vi "5.7.4-Forebrain_to_OCU-UDPServer.vi"() -> ()   [LabVIEW 2010]
doc: "Creates a named service and listens on the first available port. Whenever a client connects to the service, it responds with a message containing joystick data. The VI can be stopped using the STOP button."
uses:
  6-OCU Neurons/CommonIndicators.ctl
  4-High Neurons/4.4-How Sensor Typedef.ctl
  5.0-Global.vi
panel:
  out "5.7.2 Main Indicators":T1
  out "data out":string
  out "error out":errorcluster
  in  "error in":errorcluster
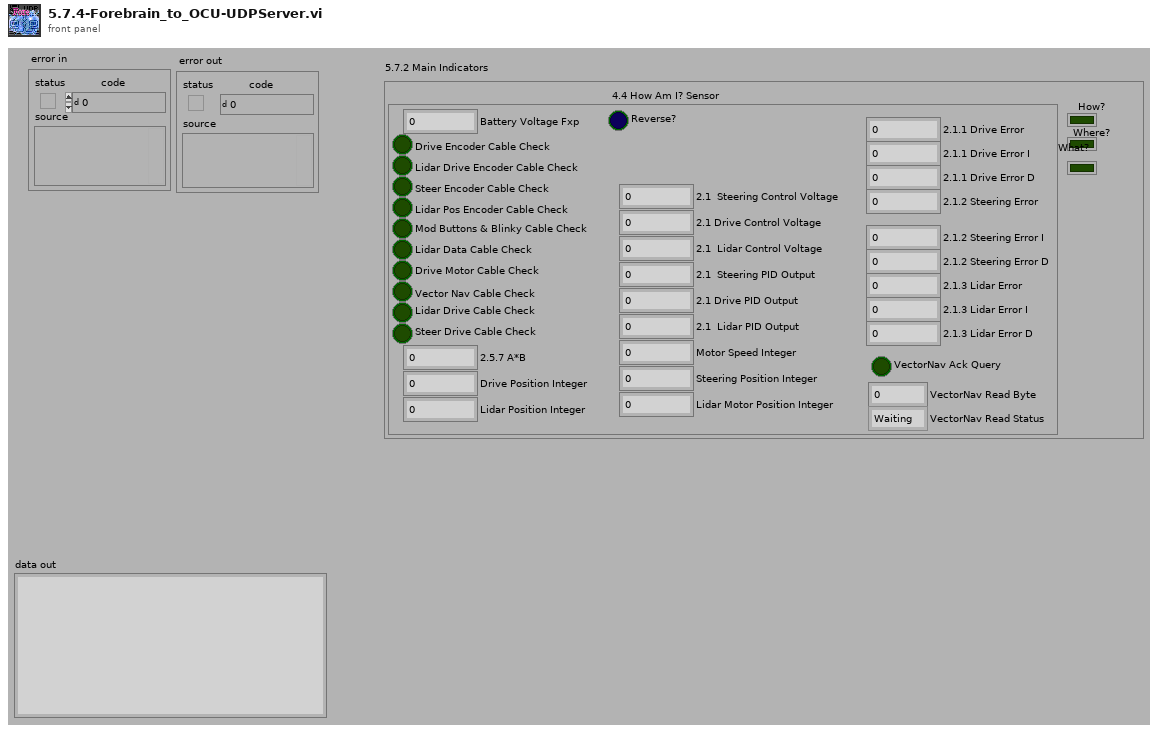
[diagram p1: front panel]
types:
  T1 = typedef "CommonIndicators.ctl" = cluster{"4.4 How Am I? Sensor":T2, "How?":bool, "Where?":bool, "What?":bool}
  T2 = typedef "4.4-How Sensor Typedef.ctl" = cluster{"Motor Speed Integer":i32, "Drive Position Integer":i32, "Lidar Position Integer":i32, "Lidar Motor Position Integer":i32, "Steering Position Integer":i32, "Battery Voltage Fxp":dbl, "Drive Encoder Cable Check":bool, "Lidar Drive Encoder Cable Check":bool, "Steer Encoder Cable Check":bool, "Lidar Pos Encoder Cable Check":bool, "Mod Buttons & Blinky Cable Check":bool, "Lidar Data Cable Check":bool, "Drive Motor Cable Check":bool, "Vector Nav Cable Check":bool, "Lidar Drive Cable Check":bool, "Steer Drive Cable Check":bool, "Reverse?":bool, "2.1  Steering Control Voltage":dbl, "2.1 Drive Control Voltage":dbl, "2.1  Lidar Control Voltage":dbl, "2.5.7 A*B":dbl, "2.1  Steering PID Output":dbl, "2.1 Drive PID Output":dbl, "2.1  Lidar PID Output":dbl, "2.1.1 Drive Error":dbl, "2.1.1 Drive Error I":dbl, "2.1.1 Drive Error D":dbl, "2.1.2 Steering Error":dbl, "2.1.2 Steering Error I":dbl, "2.1.2 Steering Error D":dbl, "2.1.3 Lidar Error":dbl, "2.1.3 Lidar Error I":dbl, "2.1.3 Lidar Error D":dbl, "VectorNav Ack Query":bool, "VectorNav Read Byte":u8, "VectorNav Read Status":enum16{"Waiting", "Reading", "Done"}}
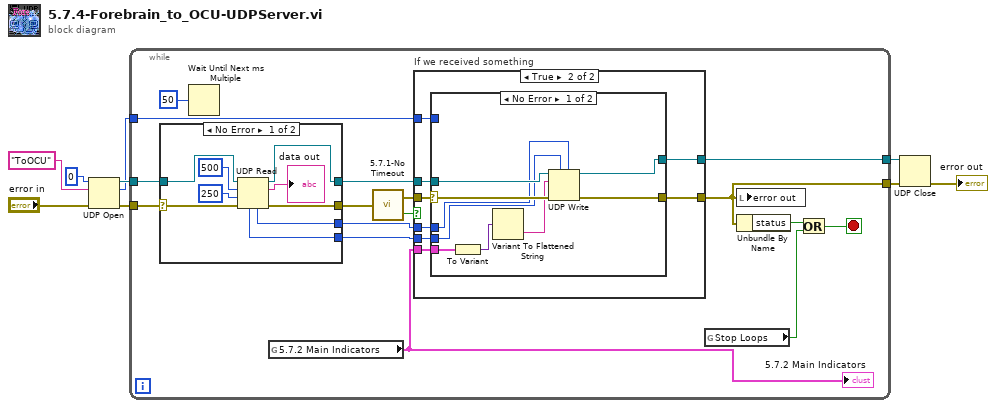
[diagram p0: block diagram]
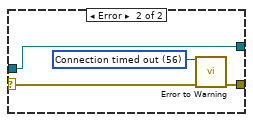
[diagram p3: hidden frame]
diagram:
  n1 = UDP Open(8:"error in", 10:"ToOCU" ("service name"), 11:u16 0 ("port")) -> (port=w8:refnum<k16>, 0:w7:errorcluster, 2:w3:u16)  [unwired: 2 in]
  n2 = while {
    tunnel: [w14] -> w5
    tunnel: w8 -> [w25]
    tunnel: w7 -> [w22]
    tunnel: [w23] -> w6
    tunnel: w3 -> [w19]
    stop <- w17 stop-if-true
    n3 = case shown="No Error" w22 {
      selector: w22 -> [w55 w58]
      tunnel: w25 -> [w57 w59]
      tunnel: [w54 w59] -> w24
      tunnel: [w53 w58] -> w13
      tunnel: [w51 _] -> w20
      tunnel: [w52 _] -> w21
      frame No Error {
        n4 = UDP Read(connection ID=w57, max size (548)=500, timeout ms (25000)=250, 8:w55) -> (data out=→"data out":string, error out=w53:errorcluster, 3:w54:refnum<k16>, 4:w51:u16, 6:w52:u32)
      }
      frame Error {
      }
    }
    n5 = Wait Until Next ms Multiple(millisecond multiple=u32 50) -> ()  [unwired: 1 out]
    n6 = global read "5.0-Global.vi" "5.7.2 Main Indicators"() -> (w11:T1)
    "5.7.2 Main Indicators" <- w11
    n7 = call "5.7.1-No Timeout.vi"("error in (no error)"=w13) -> ("No Timeout"=w15:bool, "error out"=w16:errorcluster)
    n8 = case "If we received something" shown="True" w15 {
      tunnel: w24 -> [w26 w35]
      tunnel: [w26 w34] -> w23
      tunnel: w21 -> [_ w33]
      tunnel: w20 -> [_ w32]
      tunnel: w19 -> [_ w31]
      tunnel: [w27 w30] -> w14
      tunnel: w16 -> [w27 w29]
      tunnel: w11 -> [_ w28]
      frame False {
      }
      frame True {
        n9 = case shown="No Error" w29 {
          selector: w29 -> [w44 w46]
          tunnel: w35 -> [w41 w48]
          tunnel: [w43 w45] -> w30
          tunnel: [w42 w48] -> w34
          tunnel: w33 -> [w39 _]
          tunnel: w32 -> [w40 _]
          tunnel: w31 -> [_ _]
          tunnel: w28 -> [w36 _]
          frame No Error {
            n10 = To Variant(anything=w36) -> (Variant=w38:variant)
            n11 = Variant To Flattened String(Variant=w38) -> (data string=w37:string)  [unwired: 1 out]
            n12 = UDP Write(address=w39, port or service name=w40, connection ID=w41, data in=w37, 8:w44) -> (error out=w43:errorcluster, 3:w42:refnum<k16>)  [unwired: 1 in]
          }
          frame Error {
            w47 = 56 items=["No Error", "Argument Error", "Memory Full", "Out of Zone", "End of File", "File Already Open", "Generic File IO Error", "File Not Found", "File Permission Error", "Disk Full", "Duplicate Path", "Too Many Files Open", "Not Enabled", "Resource File Not Found", "Cannot Add Resource", "Resource Not Found", "Image Not Found", "Image Memory Error", "Pen Does Not Exist", "Config Bad Type", "Config Token Not Found", "Config Parse Error", "Config Memory Error", "Bad External Code Format", "Bad External Code Offset", "External Code Not Present", "Null Window", "Destroy Window Mixup", "Null Menu", "Print Aborted", "Bad Print Record", "Print Driver Error", "Windows Error During Print", "Memory Error During Print", "Print Dialog Error", "Generic Print Error", "Invalid Device Refnum", "Device Not Found", "Device Parameter Error", "Device Unit Error", "Can't Open Device", "Device Call Aborted", "Generic Error", "Cancelled By User", "Object ID Too Low", "Object ID Too High", "Object Not In Heap", "Unknown Heap", "Bad DefProc ID", "DefProc Not In Table", "Message Out Of Range", "Null Method", "Unknown Message", "Manager Call Not Supported", "Bad address", "Connection In progress", "Connection timed out", "Connection is already in progress", "Network attribute not supported", "Network error", "Address in use", "System out of memory", "Connection aborted", "Connection refused", "Connection is not connected", "Connection is already connected", "Connection closed", "Initialize error (interapplication manager)", "Bad occurrence", "Wait on unbound occurrence handler", "Occurrence queue overflow", "Bad path", "Semaphore not signaled", "Unrecognized type (interapplication manager)"] ("1st Error to Convert")
            n13 = call <vilib>:"Error to Warning.vi"("1st Error to Convert"=w47, "error in"=w46) -> ("warning out"=w45:errorcluster)  [unwired: 13 in]
          }
        }
      }
    }
    n14 = global read "5.0-Global.vi" "Stop Loops"() -> (w12:bool)
    n15 = local write "error out"(w14) -> ()
    n16 = Unbundle By Name(w14) -> ("status"=w18:bool)
    n17 = Or(x=w18, y=w12) -> (x .or. y?=w17:bool)
  }
  n18 = UDP Close(connection ID=w6, 8:w5) -> (error out=→"error out":errorcluster)  [unwired: 1 out]
